vi "xeva-checkTemperatureSP.vi"(3 "error in (no error)":errorcluster, 4 "xeva-temperature":dbl, 5 "xeva-camref":T1) -> (0 "error out":errorcluster, 1 "xeva-temperatureSP-ok":bool)   [LabVIEW 2017]
uses:
  <vilib>/Xenics Infrared Solutions/Xeneth LabVIEW API/VIs/Controls/Camara.ctl
  <vilib>/Xenics Infrared Solutions/Xeneth LabVIEW API/Xeneth.lvlib
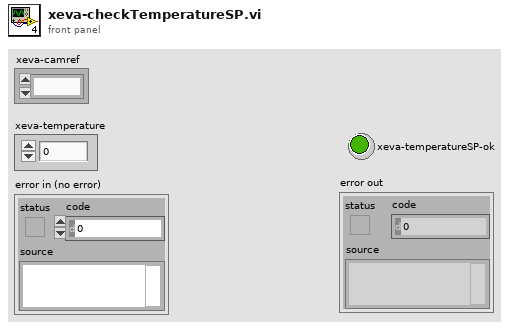
[diagram p1: front panel]
types:
  T1 = typedef "Xeneth.lvlib/Camara.ctl" = refnum<k1>
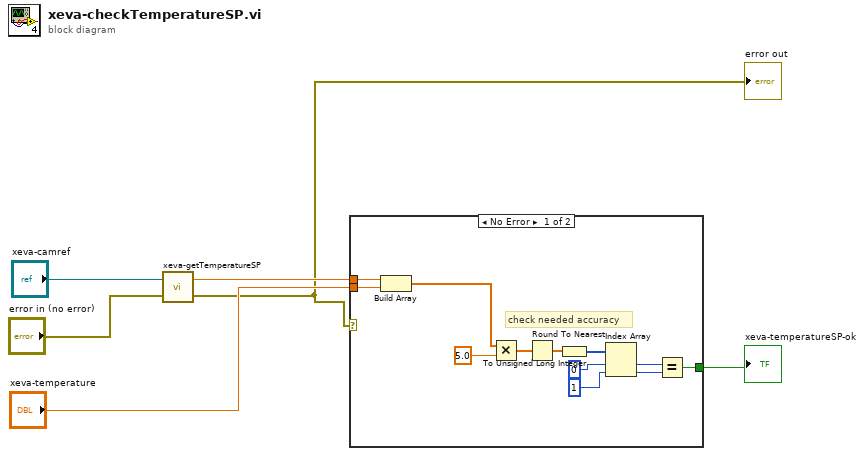
[diagram p0: block diagram]
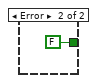
[diagram p2: hidden frame]
diagram:
  n1 = call "xeva-getTemperatureSP.vi"("error in (no error)"="error in (no error)", "xeva-camref"="xeva-camref") -> ("error out"=w1:errorcluster, "xeva-temperature-setpoint"=w4:dbl)
  "error out" <- w1
  n2 = case shown="No Error" w1 {
    tunnel: w4 -> [w16 _]
    tunnel: "xeva-temperature" -> [w15 _]
    tunnel: [w7 FALSE] -> w2
    frame No Error {
      # "check needed accuracy"
      n3 = Build Array(w16, w15) -> (w14:dbl[])
      n4 = Multiply(x=w14, y=5.0) -> (x*y=w17:dbl[])
      n5 = Round To Nearest(number=w17) -> (nearest integer value=w13:dbl[])
      n6 = To Unsigned Long Integer(number=w13) -> (unsigned 32bit integer=w12:u32[])
      n7 = Index Array(array=w12, index #1=0 ("index"), index #2=1 ("index")) -> (element #1=w8:u32, element #2=w9:u32)
      n8 = Equal?(x=w8, y=w9) -> (x = y?=w7:bool)
    }
    frame Error {
    }
  }
  "xeva-temperatureSP-ok" <- w2
